vi "ORS_AlazarDLLAcq_Xfer.vi"(8 "error in (no error)":errorcluster, 9 "#buffers":u32=1, 10 "SamplesPerBuffer":u32=65536, 11 "ATSHandle":u32=60940) -> (0 "error out":errorcluster={"status"=FALSE, "code"=5512, "source"="Abort Async Read\rATS: ApiSuccess(512)"}, 1 "Return Code":u32=589, 2 "BufferArrayOut":i16[][](array[numeric]), 3 "ATSHandleOut":u32=60940)   [LabVIEW 2024]
panel:
  out "dataB":i16[](graph)
  in  "sizeB":u32
  out "path out":path
  out "return code":i32
  out "done_records":u32
  out "dataA":i16[](graph)
  out "dt":u32=26
  in  "sizeA":u32=8192
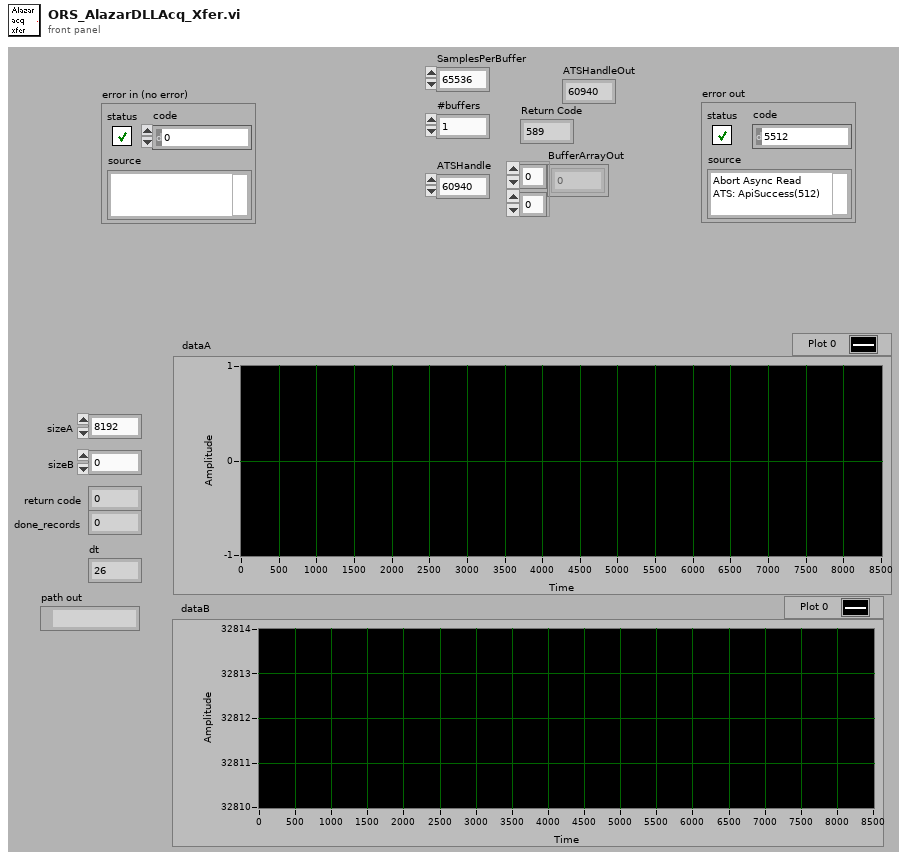
[diagram p1: front panel]
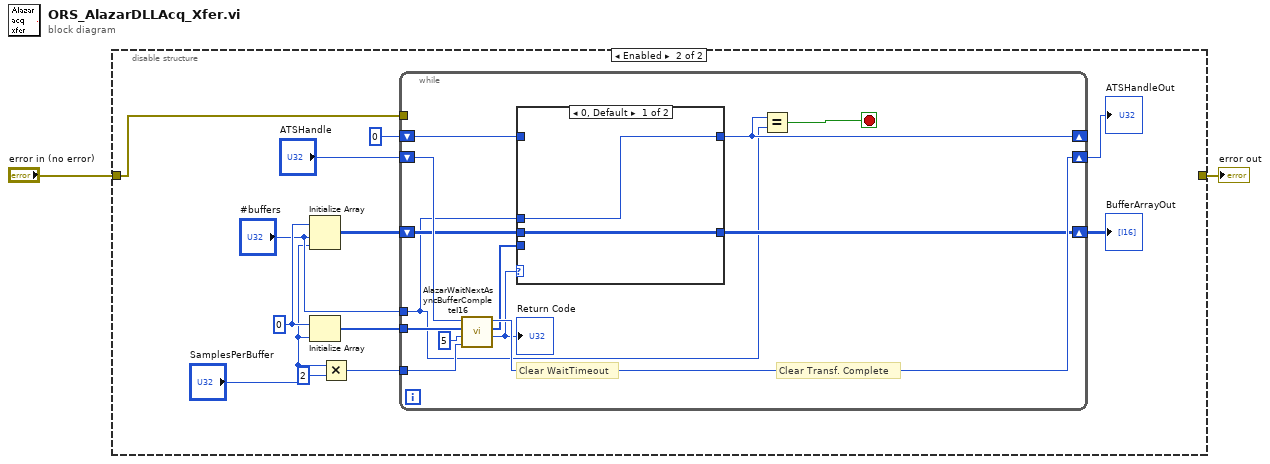
[diagram p0: block diagram]
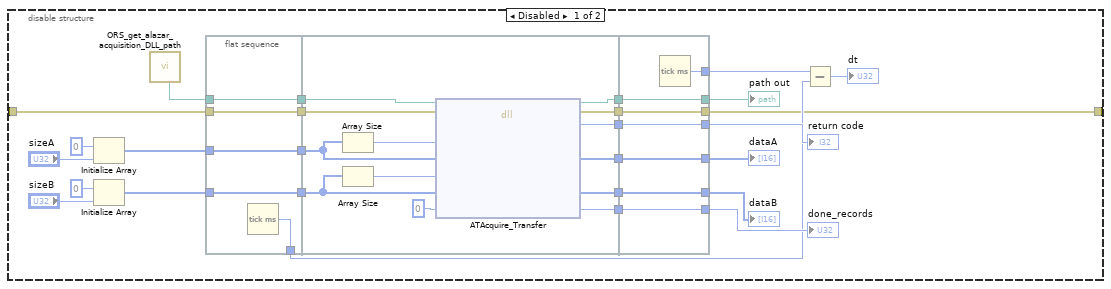
[diagram p2: hidden frame]
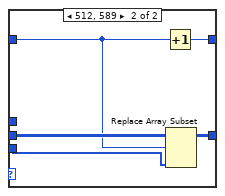
[diagram p3: hidden frame]
diagram:
  n1 = disable-structure shown="Enabled" {
    disable-tunnel: "error in (no error)" -> [w4 w65]
    disable-tunnel: [w3 _] -> w1
    frame Disabled {
      n2 = Initialize Array(i16 0 ("element"), "sizeA") -> (w16:i16[])
      n3 = Initialize Array(i16 0 ("element"), "sizeB") -> (w7:i16[])
      n4 = call "ORS_get_alazar_acquisition_DLL_path.vi"() -> ("Alazar Acquisition DLL path"=w5:path)  [unwired: 10 in, 1 out]
      n5 = flat-sequence {
        tunnel: w5 -> [w33]
        tunnel: w16 -> [w34]
        tunnel: [w34] -> w29
        tunnel: [w33] -> w28
        tunnel: [w32] -> w13
        tunnel: w7 -> [w31]
        tunnel: [w31] -> w27
        tunnel: [w30] -> w26
        tunnel: w4 -> [w30]
        tunnel: [w47] -> w25
        tunnel: [w41] -> w24
        tunnel: [w43] -> w23
        tunnel: w29 -> [w40]
        tunnel: w28 -> [w44]
        tunnel: [w42] -> w22
        tunnel: w27 -> [w39]
        tunnel: [w37] -> w21
        tunnel: w26 -> [w36]
        tunnel: [w35] -> w20
        tunnel: [w52] -> w14
        tunnel: [w53] -> w15
        tunnel: [w54] -> w18
        tunnel: w25 -> [w54]
        tunnel: w24 -> [w53]
        tunnel: w23 -> [w52]
        tunnel: [w51] -> w12
        tunnel: [w50] -> w10
        tunnel: w22 -> [w50]
        tunnel: [w49] -> w6
        tunnel: w21 -> [w49]
        tunnel: [w48] -> w3
        tunnel: w20 -> [w48]
        frame #0 {
          n6 = Tick Count (ms)() -> (millisecond timer value=w32:u32)
        }
        frame #1 {
          n7 = Array Size(array=w40) -> (size(s)=w46:i32)
          n8 = Array Size(array=w39) -> (size(s)=w38:i32)
          n9 = dll-call lib="Z:/Software/AlazarTech/ATS-SDK/5.6.3/ATS9462-SDK/Dual Port Async/C/PostBuffer_Recommended/at_acquire/Release/at_acquire.dll" fn="ATAcquire_Transfer" ("at_acquire.dll:TestFunc")(path in=w44, error in=w36, "sizeA"=w46, "dataA"=w40, "sizeB"=w38, "dataB"=w39, "done_records"=u32 0) -> (path out=w42:path, error out=w35:errorcluster, "return type"=w47:i32, "dataA"=w41:i16[], "dataB"=w37:i16[], "done_records"=w43:u32)  [unwired: 3 in]
        }
        frame #2 {
          n10 = Tick Count (ms)() -> (millisecond timer value=w51:u32)
        }
      }
      n11 = Subtract(x=w12, y=w13) -> (x-y=→"dt":u32)
      "return code" <- w18
      "done_records" <- w14
      "dataA" <- w15
      "path out" <- w10
      "dataB" <- w6
    }
    frame Enabled {
      w63 = i16 0 ("element")
      n12 = Initialize Array(w63, "#buffers", "SamplesPerBuffer") -> (w64:i16[][])
      n13 = Initialize Array(w63, "SamplesPerBuffer") -> (w62:i16[])
      n14 = Multiply(x="SamplesPerBuffer", y=u32 2) -> (x*y=w55:u32)
      n15 = while {
        tunnel: w65 -> [_]
        shift-right: [w78] -> w60
        shift-left: "ATSHandle" -> [w79]
        shift-right: [w73] -> w59
        shift-left: w64 -> [w75]
        tunnel: w62 -> [w76]
        shift-right: [w69] -> _
        shift-left: 0 -> [w74]
        tunnel: "#buffers" -> [w67]
        tunnel: w55 -> [w68]
        stop <- w70 stop-if-true
        # "Clear Transf. Complete"
        # "Clear WaitTimeout"
        n16 = call "AlazarWaitNextAsyncBufferCompleteI16.vi"("bytesToCopy"=w68, "timeout_ms"=u32 5, "Buffer"=w76, "Handle"=w79) -> ("Return Code"=w71:u32, "Buffer"=w72:u16[], "Handle"=w78:u32)  [unwired: 1 in]
        "Return Code" <- w71
        n17 = case shown="0, Default" w71 {
          tunnel: w75 -> [w81 w86]
          tunnel: w74 -> [_ w85]
          tunnel: [w80 w84] -> w69
          tunnel: [w81 w83] -> w73
          tunnel: w72 -> [_ w82]
          tunnel: w67 -> [w80 _]
          frame 0, Default {
          }
          frame 512, 589 {
            n18 = Increment(x=w85) -> (x+1=w84:u32)
            n19 = Replace Array Subset(array=w86, new element=w82, index (row)=w85) -> (w83:i16[][])  [unwired: 1 in]
          }
        }
        n20 = Equal?(x=w69, y=w67) -> (x = y?=w70:bool)
      }
      "ATSHandleOut" <- w60
      "BufferArrayOut" <- w59
    }
  }
  "error out" <- w1
